vi "Update.vi"(0 "reference in":refnum<class "Proccess.lvclass">, 11 "error in (no error)":errorcluster) -> (4 "reference out":refnum<class "Proccess.lvclass">, 15 "error out":errorcluster)   [LabVIEW 2019, in "Proccess.lvclass"]
uses:
  Proccess.lvclass
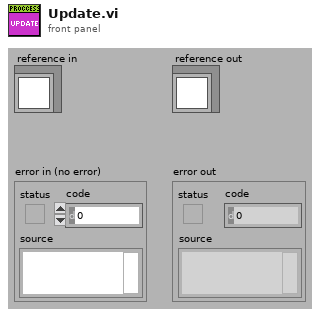
[diagram p1: front panel]
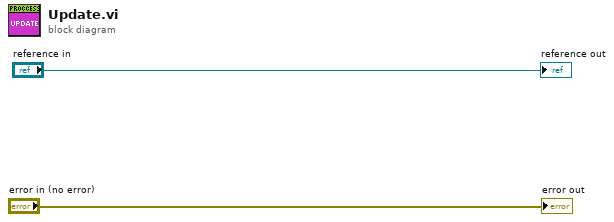
[diagram p0: block diagram]
diagram:
  "error out" <- "error in (no error)"
  "reference out" <- "reference in"
